vi "test_scanEngineCore.vi"() -> ()   [LabVIEW 2016]
uses:
  <vilib>/rvi/DesktopExecutionNode/Execution/niFpgaDEN_Execute.vi
  <vilib>/rvi/DesktopExecutionNode/DesktopExecutionNode.xnode
panel:
  in  "stop":bool
  out "pixelCount":i32
  in  "lower limit":i32
  in  "upper limit":i32
  out "simulationProgressDone":dbl(slide) scale=0.0..1.0
  out "fastIndices":cluster{"index":u16, "next":u16}[](array[cluster])
  out "debugIndices":T1(array[cluster])
  out "XY Graph":cluster{i32[], i16[]}[](graph)
  out "outputValid":cluster{"scanValid":bool, "slowValid":bool}[](array[cluster])
  in  "scanOffset":cluster{"x":fxp<+/-,16,1>, "y":fxp<+/-,16,1>}
  out "slowMoving":bool[](array[boolean])
  out "output":T2(array[cluster])
  out "clocks":T3(array[cluster])
  out "savedPoint":T4(array[cluster])
  out "slowIndices":cluster{"index":u16, "f":u16}[](array[cluster])
  in  "singleDirectionScan":bool=TRUE
  in  "moveToPoint":cluster{"x":fxp<+/-,16,1>, "y":fxp<+/-,16,1>}
  in  "moveRates":T5={"moveToDecFactor"=5, "moveToWaveSize"=128}
  in  "scanRates":T6={"outputRate"=3, "fastDecFactor"=4, "outWaveSizeFast"=128, "pplUpsampling"=8, "numLines"=16}
  in  "scanSize":T7={"fastScanSize"=0.5, "slowScanSize"=0.5}
  in  "scanTurnOnTime":i32
  in  "simulationTime":i32
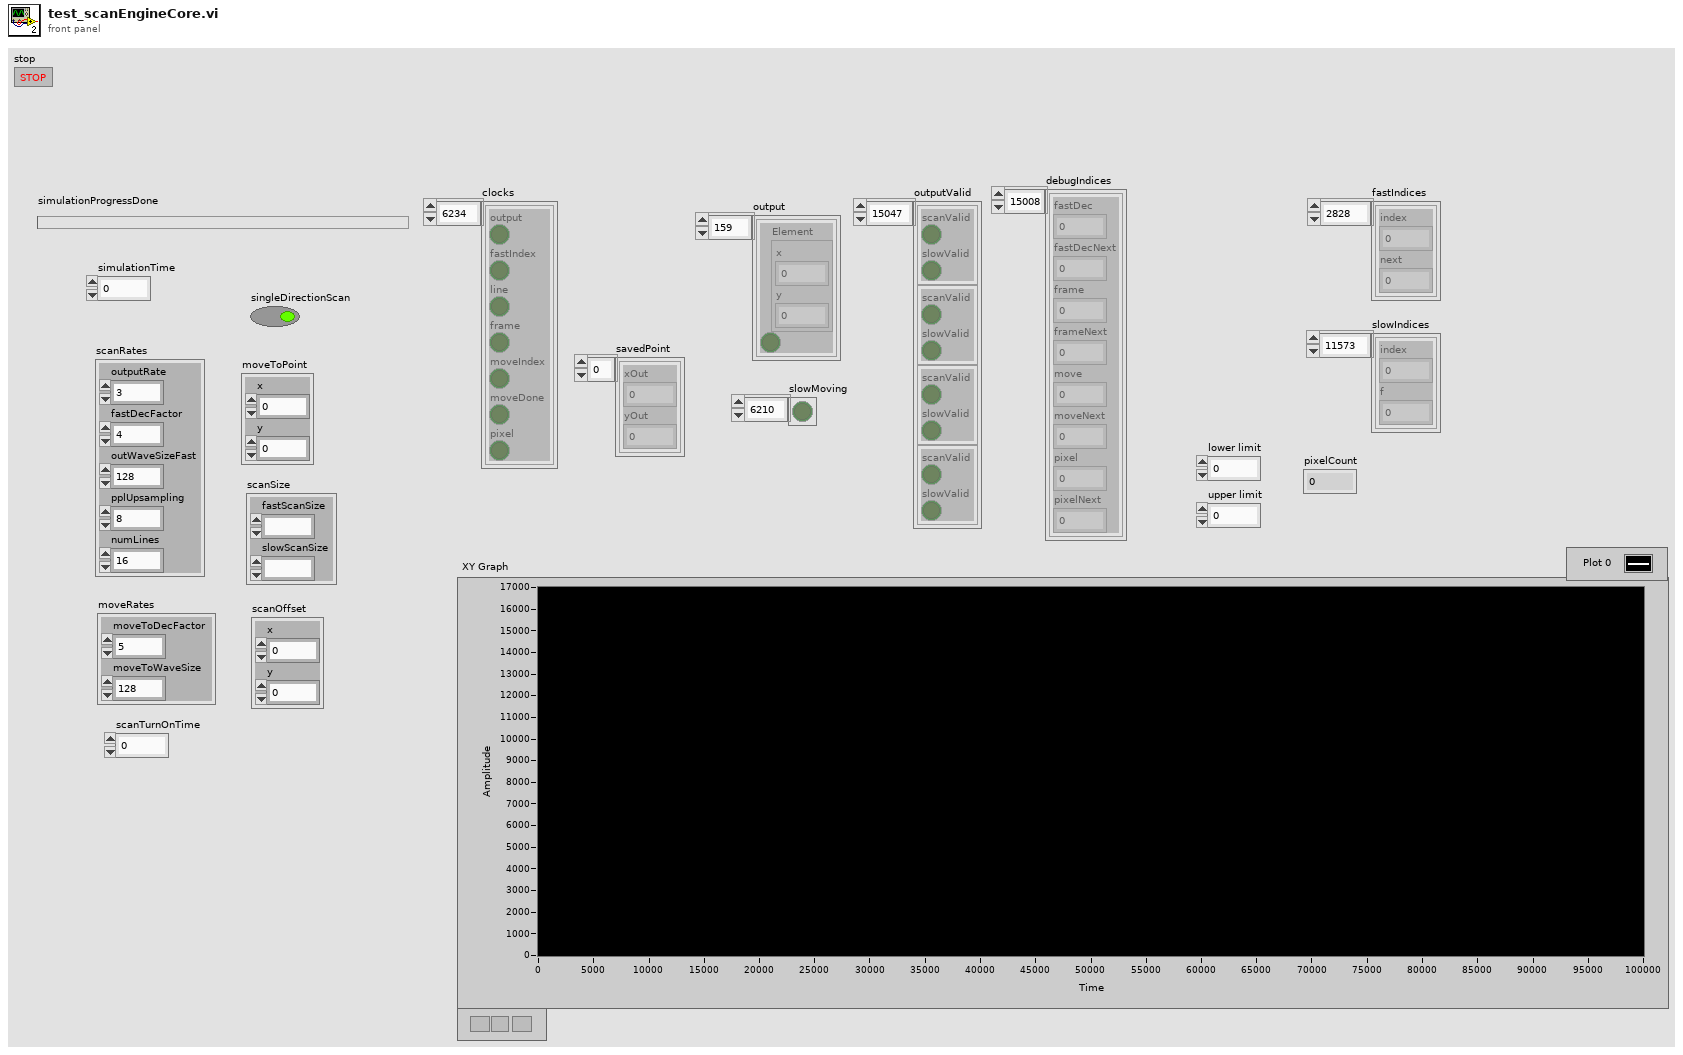
[diagram p1: front panel]
types:
  T1 = cluster{"fastDec":u16, "fastDecNext":u16, "frame":u16, "frameNext":u16, "move":u16, "moveNext":u16, "pixel":u16, "pixelNext":u16}[]
  T2 = cluster{"Element":cluster{"x":i16, "y":i16}, bool}[]
  T3 = cluster{"output":bool, "fastIndex":bool, "line":bool, "frame":bool, "moveIndex":bool, "moveDone":bool, "pixel":bool}[]
  T4 = cluster{"xOut":fxp<+/-,18,2>, "yOut":fxp<+/-,18,2>}[]
  T5 = cluster{"moveToDecFactor":u16, "moveToWaveSize":u16}
  T6 = cluster{"outputRate":u16, "fastDecFactor":u16, "outWaveSizeFast":u16, "pplUpsampling":u16, "numLines":u16}
  T7 = cluster{"fastScanSize":fxp<+,17,1>, "slowScanSize":fxp<+,17,1>}
  T8 = cluster{"a":fxp<+/-,18,2>, "b":fxp<+/-,18,2>, "c":fxp<+/-,18,2>, "d":fxp<+/-,18,2>}
  T9 = cluster{"xOut":fxp<+/-,18,2>, "yOut":fxp<+/-,18,2>}
  T10 = cluster{"output":bool, "fastIndex":bool, "line":bool, "frame":bool, "moveIndex":bool, "moveDone":bool, "pixel":bool}
  T11 = cluster{"Element":cluster{"x":i16, "y":i16}, bool}
  T12 = cluster{"fastDec":u16, "fastDecNext":u16, "frame":u16, "frameNext":u16, "move":u16, "moveNext":u16, "pixel":u16, "pixelNext":u16}
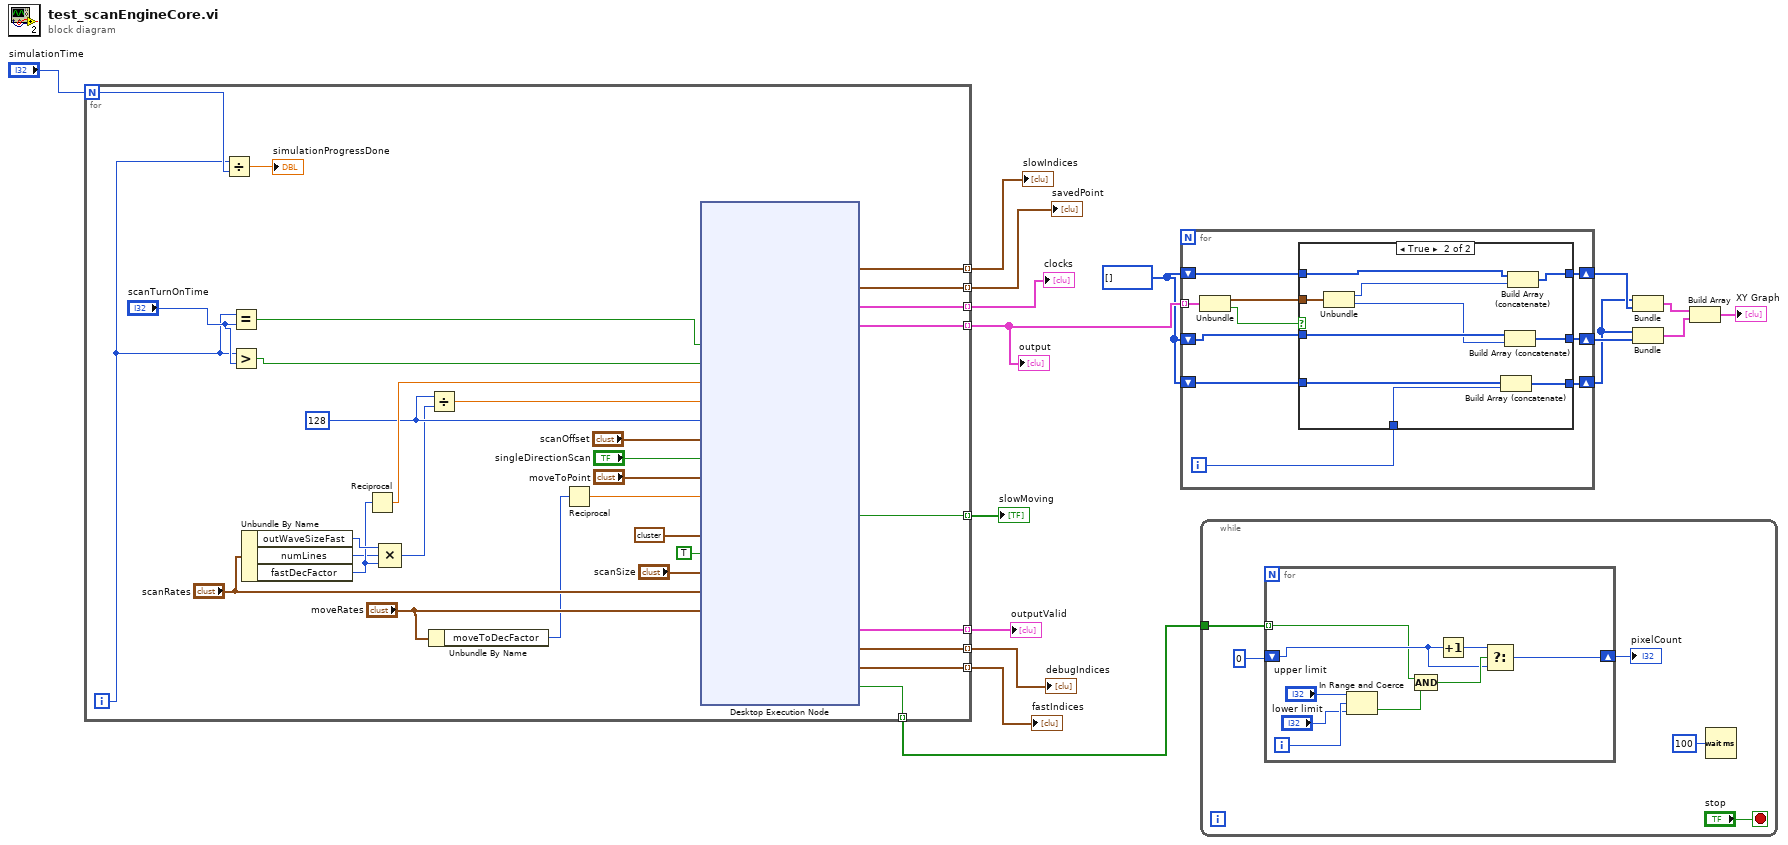
[diagram p0: block diagram]
diagram:
  w3 = i16[] []
  n1 = for {
    N: "simulationTime" -> [w21]
    tunnel: [w46] -> w13 mode=indexing
    tunnel: [w45] -> w2 mode=indexing
    tunnel: [w44] -> w15 mode=indexing
    tunnel: [w43] -> w16 mode=indexing
    tunnel: [w42] -> w14 mode=indexing
    tunnel: [w24] -> w12 mode=indexing
    tunnel: [w23] -> w6 mode=indexing
    tunnel: [w22] -> w5 mode=indexing
    tunnel: [w18] -> w1 mode=indexing
    i -> [w20]
    w31 = u16 128 ("outWaveSizeSlow")
    n2 = Divide(x=w20, y=w21) -> (x/y=→"simulationProgressDone":dbl)
    n3 = Equal?(x=w20, y="scanTurnOnTime") -> (x = y?=w41:bool)
    n4 = Greater?(x=w20, y="scanTurnOnTime") -> (0:w39:bool)
    n5 = Unbundle By Name("scanRates") -> ("outWaveSizeFast"=w34:u16, "numLines"=w32:u16, "fastDecFactor"=w33:u16)
    n6 = Reciprocal(x=w33) -> (1/x=w35:dbl)
    n7 = Compound Arithmetic op=MULTIPLY(w34, w32, w33) -> (w30:u16)
    n8 = Divide(x=w31, y=w30) -> (x/y=w29:dbl)
    n9 = Unbundle By Name("moveRates") -> ("moveToDecFactor"=w27:u16)
    n10 = Reciprocal(x=w27) -> (1/x=w26:dbl)
    n11 = xnode "Desktop Execution Node"("doSlowMoveFIFO"=w41, "scanEnabled"=w39, "fastDecFactorInv"=w35, "slowUpStep"=w29, "outWaveSizeSlow"=w31, "scanOffset"="scanOffset", "singleDirectionScan"="singleDirectionScan", "moveToPoint"="moveToPoint", "invMoveToDec"=w26, "outputMatrix"=T8 {"a"=1.0, "b"=0.0, "c"=0.0, "d"=1.0}, "frioRecordingEnable"=TRUE, "scanSize"="scanSize", "scanRates"="scanRates", "moveRates"="moveRates") -> ("slowIndices"=w43:cluster{"index":u16, "f":u16}, "savedPoint"=w44:T9, "clocks"=w45:T10, "output"=w46:T11, "slowMoving"=w42:bool, "outputValid"=w24:cluster{"scanValid":bool, "slowValid":bool}, "indices"=w23:T12, "fastIndices"=w22:cluster{"index":u16, "next":u16}, "pixelEvent"=w18:bool)  [unwired: 1 in, 1 out]
  }
  "slowIndices" <- w16
  "savedPoint" <- w15
  "clocks" <- w2
  "output" <- w13
  "slowMoving" <- w14
  "outputValid" <- w12
  "debugIndices" <- w6
  "fastIndices" <- w5
  n12 = for {
    tunnel: w13 -> [w59] mode=indexing
    shift-right: [w57] -> w11
    shift-left: w3 -> [w58]
    shift-right: [w52] -> w10
    shift-left: w3 -> [w53]
    shift-right: [w51] -> w9
    shift-left: w3 -> [w50]
    i -> [w54]
    n13 = Unbundle(w59) -> ("Element"=w55:cluster{"x":i16, "y":i16}, w56:bool)
    n14 = case shown="True" w56 {
      tunnel: w58 -> [w62 w71]
      tunnel: [w62 w70] -> w57
      tunnel: w55 -> [_ w72]
      tunnel: w54 -> [_ w65]
      tunnel: w53 -> [w60 w69]
      tunnel: [w60 w68] -> w52
      tunnel: [w61 w64] -> w51
      tunnel: w50 -> [w61 w63]
      frame False {
      }
      frame True {
        n15 = Unbundle(w72) -> ("x"=w67:i16, "y"=w66:i16)
        n16 = Build Array (concatenate)(w63, w65) -> (w64:i32[])
        n17 = Build Array (concatenate)(w69, w66) -> (w68:i16[])
        n18 = Build Array (concatenate)(w71, w67) -> (w70:i16[])
      }
    }
  }
  n19 = while {
    tunnel: w1 -> [w75]
    stop <- "stop" stop-if-true
    n20 = for {
      shift-right: [w79] -> w76
      shift-left: 0 -> [w81]
      tunnel: w75 -> [w78] mode=indexing
      i -> [w86]
      n21 = In Range and Coerce(upper limit="upper limit", x=w86, lower limit="lower limit") -> (In Range?=w85:bool)  [unwired: 1 out]
      n22 = Compound Arithmetic op=AND(w78, w85) -> (w82:bool)
      n23 = Increment(x=w81) -> (x+1=w80:i32)
      n24 = Select(t=w80, s=w82, f=w81) -> (s? t:f=w79:i32)
    }
    "pixelCount" <- w76
    n25 = Wait (ms)(milliseconds to wait=u32 100) -> ()  [unwired: 1 out]
  }
  n26 = Bundle(w9, w11) -> (w8:cluster{i32[], i16[]})  [unwired: 1 in]
  n27 = Bundle(w9, w10) -> (w4:cluster{i32[], i16[]})  [unwired: 1 in]
  n28 = Build Array(w8, w4) -> (→"XY Graph":cluster{i32[], i16[]}[])
